vi "Test Step Menu Items.vi"() -> (3 "Array":string[][](array[string])=[["NI_Flow_If", "Flow Control"], ["NI_Flow_For", "Flow Control"], ["NI_Flow_End", "Flow Control"], ["LV_Send_Command", "Commands"], ["LV_Check_Command", "Commands"], ["LV_Test_Value", "Tests"], ["LV_Value_Above", "Tests"], ["LV_Value_Below", "Tests"]])   [LabVIEW 2020]
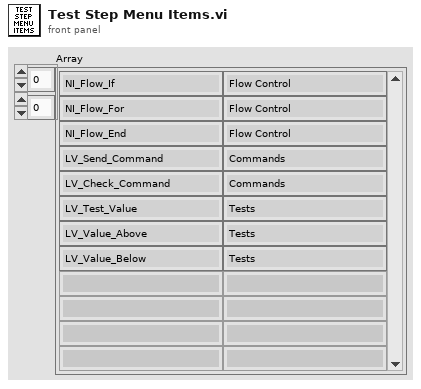
[diagram p1: front panel]
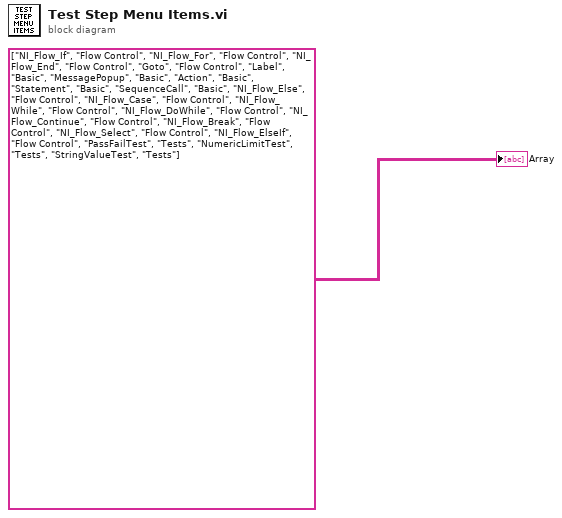
[diagram p0: block diagram]
diagram:
  "Array" <- string[][] [["NI_Flow_If", "Flow Control"], ["NI_Flow_For", "Flow Control"], ["NI_Flow_End", "Flow Control"], ["Goto", "Flow Control"], ["Label", "Basic"], ["MessagePopup", "Basic"], ["Action", "Basic"], ["Statement", "Basic"], ["SequenceCall", "Basic"], ["NI_Flow_Else", "Flow Control"], ["NI_Flow_Case", "Flow Control"], ["NI_Flow_While", "Flow Control"], ["NI_Flow_DoWhile", "Flow Control"], ["NI_Flow_Continue", "Flow Control"], ["NI_Flow_Break", "Flow Control"], ["NI_Flow_Select", "Flow Control"], ["NI_Flow_ElseIf", "Flow Control"], ["PassFailTest", "Tests"], ["NumericLimitTest", "Tests"], ["StringValueTest", "Tests"]]
